vi "Write Offset.vi"(8 "error in (no error)":errorcluster, 10 "Offset":i32, 11 "CAN_RW_CORE in":refnum<class "L2ENET_RW_CORE.lvclass">) -> (0 "error out":errorcluster, 3 "CAN_RW_CORE out":refnum<class "L2ENET_RW_CORE.lvclass">)   [LabVIEW 2021, in "L2ENET_RW_CORE.lvclass"]
uses:
  L2ENET_RW_CORE.lvclass
  L2ENET_RW_CORE.lvclass/L2ENET_RW_CORE.ctl
  <vilib>/CIF Foundation/CIF PCAP Parse and Build/pcap_Parse_Build_CIF.lvclass
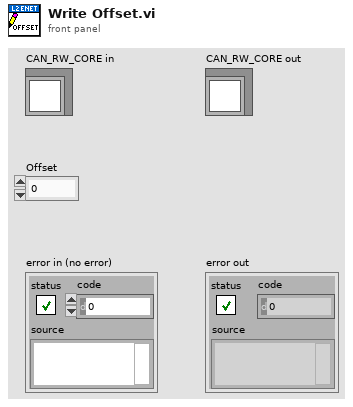
[diagram p1: front panel]
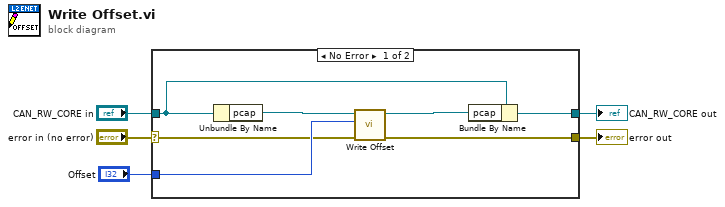
[diagram p0: block diagram]
diagram:
  n1 = case shown="No Error" "error in (no error)" {
    selector: "error in (no error)" -> [w7 w13]
    tunnel: [w6 w13] -> w4
    tunnel: [w12 w14] -> w2
    tunnel: "CAN_RW_CORE in" -> [w10 w14]
    tunnel: "Offset" -> [w11 _]
    frame No Error {
      n2 = Unbundle By Name(w10) -> ("pcap"=w9:refnum<class "pcap_Parse_Build_CIF.lvclass">)
      n3 = call <vilib>:"Write Offset.vi"("error in (no error)"=w7, "Offset"=w11, "pcap Parse and Build in"=w9) -> ("error out"=w6:errorcluster, "pcap Parse and Build out"=w8:refnum<class "pcap_Parse_Build_CIF.lvclass">)  [unwired: 7 in]
      n4 = Bundle By Name(cluster=w10, "pcap"=w8) -> (w12:refnum<class "L2ENET_RW_CORE.lvclass">)
    }
    frame Error {
    }
  }
  "error out" <- w4
  "CAN_RW_CORE out" <- w2
